vi "sub_FPGATOHOST Voltage.vi"(1 "Input":i16) -> (0 "Output":dbl)   [LabVIEW 2015]
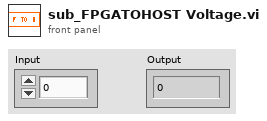
[diagram p1: front panel]
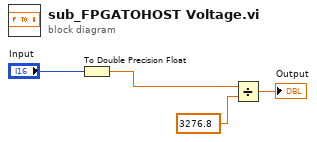
[diagram p0: block diagram]
diagram:
  n1 = To Double Precision Float(number="Input") -> (double precision float=w1:dbl)
  n2 = Divide(x=w1, y=3276.8) -> (x/y=→"Output":dbl)
